vi "LUCS001RT_UBx_RS232_ClearFIFO.vi"(8 "error in":errorcluster, 9 "FPGA VI Reference":T1) -> (0 "error out":errorcluster, 1 "FPGA VI Reference Out":T1)   [LabVIEW 2020]
uses:
  <vilib>/rvi/interface/nirviMethod/nirviMethod.xnode
  SourceCodeFPGA/LUCS001_UBx_RS232_ReadMessage.vi
  SourceCode_Host/FPGA Bitfiles/LUCS001h.lvproj_FPGA Target 1_LUCS001_UBx_RS232_~2D.lvbit
  <vilib>/rvi/errors/niLvFpgaMergeErrorWithErrorCode.vi
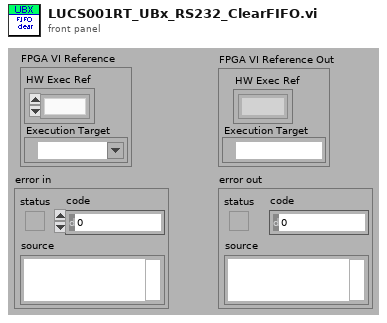
[diagram p1: front panel]
types:
  T1 = cluster{"HW Exec Ref":refnum<k1>, "Execution Target":refnum<visa-resource-name>}
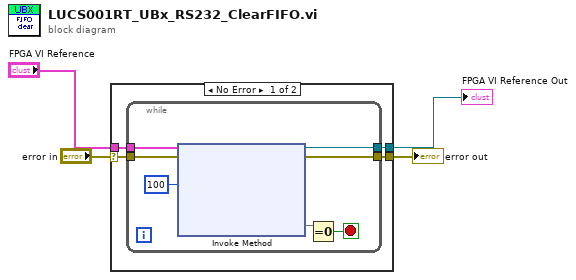
[diagram p0: block diagram]
diagram:
  n1 = case shown="No Error" "error in" {
    selector: "error in" -> [w5 w16]
    tunnel: [w8 _] -> w1
    tunnel: "FPGA VI Reference" -> [w7 _]
    tunnel: [w6 w16] -> w4
    frame No Error {
      n2 = while {
        tunnel: w5 -> [w15]
        tunnel: [w14] -> w6
        tunnel: w7 -> [w13]
        tunnel: [w12] -> w8
        stop <- w9 stop-if-true
        n3 = xnode "Invoke Method"("FPGA VI Reference In"=w13, "error in"=w15, "Number of Elements"=u32 100) -> ("FPGA VI Reference Out"=w12:refnum<k20>, "error out"=w14:errorcluster, "Elements Remaining"=w10)  [unwired: 1 in, 1 out]
        n4 = Equal To 0?(x=w10) -> (x = 0?=w9:bool)
      }
    }
    frame Error {
    }
  }
  "error out" <- w4
  "FPGA VI Reference Out" <- w1
